vi "SPI9910.vi"(0 "Port In":refnum<visa-resource-name>, 1 "Register":u8, 2 "Input":u8[](array[numeric]), 3 "Offset":u8, 4 "Command":u32(ring) items=["Write", "Update", "Read"]) -> (5 "Port Out":refnum<visa-resource-name>, 6 "Output":u8[](array[numeric]))   [LabVIEW 2014]
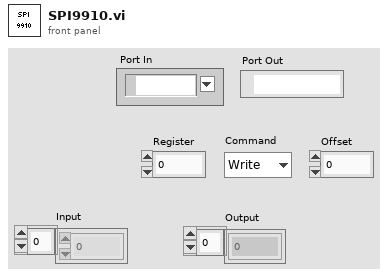
[diagram p1: front panel]
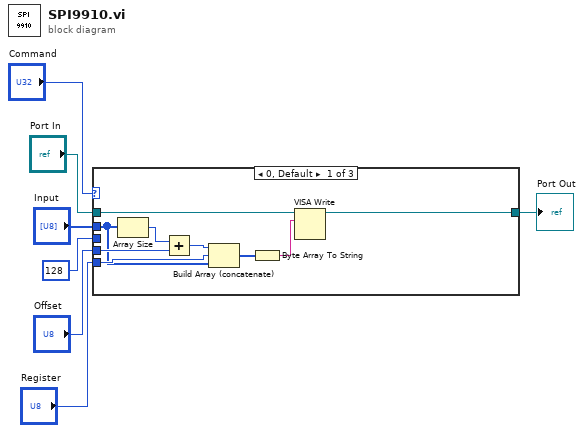
[diagram p0: block diagram]
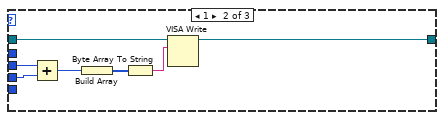
[diagram p2: hidden frame]
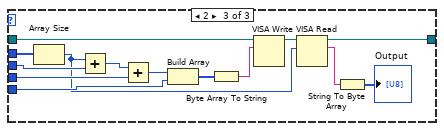
[diagram p3: hidden frame]
diagram:
  n1 = case shown="0, Default" "Command" {
    tunnel: "Port In" -> [w16 w19 w32]
    tunnel: "Input" -> [w9 _ w26]
    tunnel: "Register" -> [w15 _ w34]
    tunnel: "Offset" -> [w13 w23 w35]
    tunnel: u8 128 ("x") -> [_ w18 w28]
    tunnel: [w8 w17 w24] -> w1
    frame 0, Default {
      n2 = Array Size(array=w9) -> (size(s)=w14:i32)
      n3 = Add(x=w14, y=w13) -> (x+y=w12:i32)
      n4 = Build Array (concatenate)(w12, w15, w9) -> (w11:i32[])
      n5 = Byte Array To String(unsigned byte array=w11) -> (string=w10:string)
      n6 = VISA Write(VISA resource name=w16, write buffer=w10) -> (VISA resource name out=w8:refnum<visa-resource-name>)  [unwired: 1 in, 2 out]
    }
    frame 1 {
      n7 = Add(x=w18, y=w23) -> (x+y=w22:u8)
      n8 = Build Array(w22) -> (w21:u8[])
      n9 = Byte Array To String(unsigned byte array=w21) -> (string=w20:string)
      n10 = VISA Write(VISA resource name=w19, write buffer=w20) -> (VISA resource name out=w17:refnum<visa-resource-name>)  [unwired: 1 in, 2 out]
    }
    frame 2 {
      n11 = Array Size(array=w26) -> (size(s)=w25:i32)
      n12 = Add(x=w25, y=w28) -> (x+y=w27:i32)
      n13 = Add(x=w27, y=w35) -> (x+y=w37:i32)
      n14 = Build Array(w37, w34) -> (w36:i32[])
      n15 = Byte Array To String(unsigned byte array=w36) -> (string=w33:string)
      n16 = VISA Write(VISA resource name=w32, write buffer=w33) -> (VISA resource name out=w31:refnum<visa-resource-name>)  [unwired: 1 in, 2 out]
      n17 = VISA Read(VISA resource name=w31, byte count=w25) -> (VISA resource name out=w24:refnum<visa-resource-name>, read buffer=w30:string)  [unwired: 1 in, 2 out]
      n18 = String To Byte Array(string=w30) -> (unsigned byte array=→"Output":u8[])
    }
  }
  "Port Out" <- w1
